vi "LED_Green.vi"(9 "inten":dbl=4.16) -> ()   [LabVIEW 2012]
panel:
  in  "Green":tag[](array[tag])
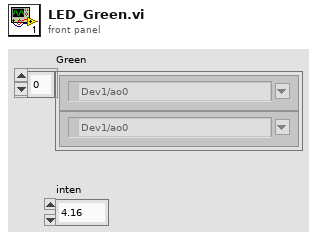
[diagram p1: front panel]
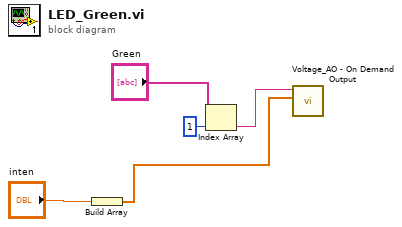
[diagram p0: block diagram]
diagram:
  n1 = Build Array("inten") -> (w1:dbl[])
  n2 = Index Array(array="Green", index=1) -> (element=w3:tag)
  n3 = call "Voltage_AO - On Demand Output.vi"("Output Array"=w1, "Physical Channel(s)"=w3) -> ()  [unwired: 10 in]
